vi "FTW-JSON-RegexHeader.vi"(1 "Regular Expression Body":string) -> (0 "Regular Expression with Header":string)   [LabVIEW 2014]
panel:
  # "Inputs"
  # "Outputs"
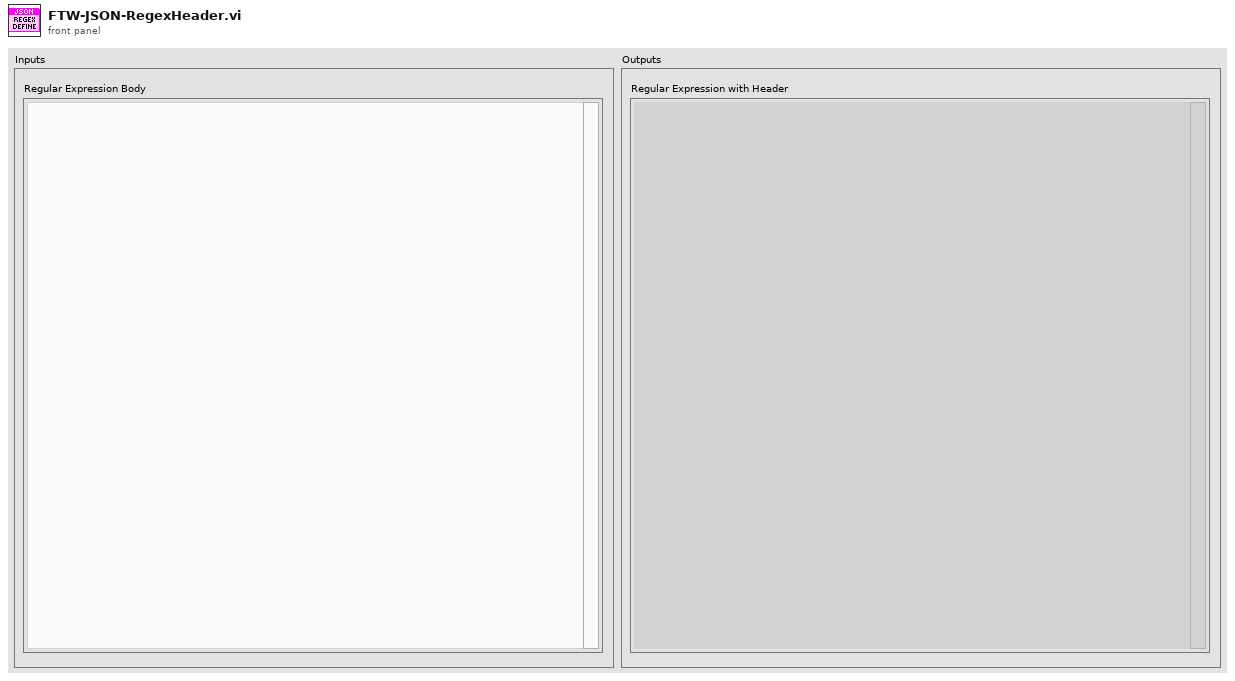
[diagram p1: front panel]
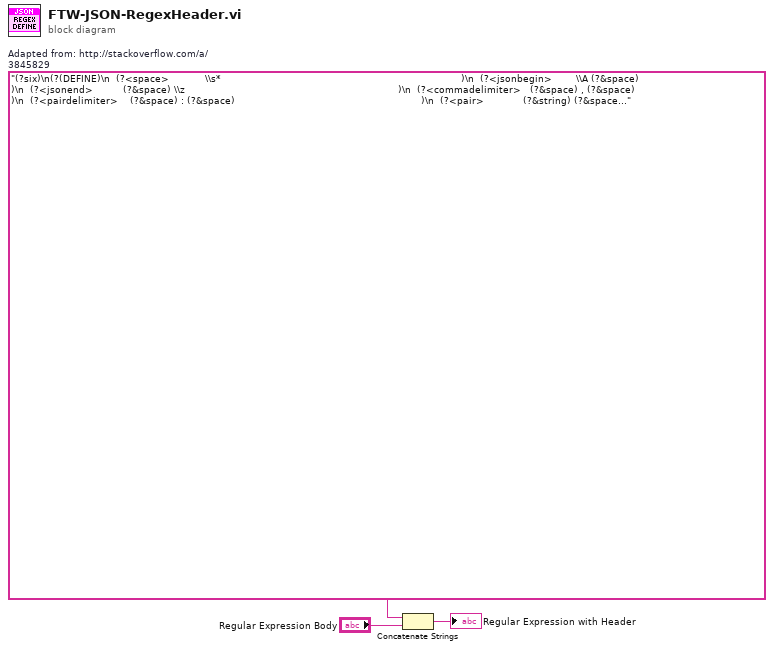
[diagram p0: block diagram]
diagram:
  w3 = "(?six)\n(?(DEFINE)\n  (?<space>            \\s*                                                                                )\n  (?<jsonbegin>        \\A (?&space)                                                                       )\n  (?<jsonend>          (?&space) \\z                                                                       )\n  (?<commadelimiter>   (?&space) , (?&space)                                                              )\n  (?<pairdelimiter>    (?&space) : (?&space)                                                              )\n  (?<pair>             (?&string) (?&space) : (?&space) (?&element)                                       )\n  (?<ftwpair>          (?&string) (?&space) : (?&space) (?&ftwelement)                                    )\n  (?<arrayelement>     (?&space) (?&element) (?&space)                                                    )\n  (?<number>           -? (?=[1-9]|0(?!\\d)) \\d+ (?:\\.\\d+)? (?:[eE][+-]?\\d+)?                              )\n  (?<ftwhexnum>        0x[0-9A-F]{2,16}                                                                   )\n  (?<boolean>          true | false                                                                       )\n  (?<null>             null                                                                               )\n  (?<stringinner>      (?:[^\"\\\\\\b\\f\\n\\r\\t] | \\\\[\"\\\\bfnrt\\/] | \\\\u[0-9a-f]{4})*                            )\n  (?<string>           \\\" (?&stringinner) \\\"                                                              )\n  (?<objectopen>       \\{ (?&space)                                                                       )\n  (?<arrayopen>        \\[ (?&space)                                                                       )\n  (?<objectclose>      (?&space) \\}                                                                       )\n  (?<arrayclose>       (?&space) \\]                                                                       )\n  (?<objectbegin>      (?&jsonbegin) (?&objectopen)                                                       )\n  (?<arraybegin>       (?&jsonbegin) (?&arrayopen)                                                        )\n  (?<objectend>        (?&objectclose) (?&jsonend)                                                        )\n  (?<arrayend>         (?&arrayclose)  (?&jsonend)                                                        )\n  (?<objectinner>      (?:(?&pair)    (?:(?&commadelimiter) (?&pair))*)?                                  )\n  (?<ftwobjectinner>   (?:(?&ftwpair) (?:(?&commadelimiter) (?&ftwpair))*)?                               )\n  (?<arrayinner>       (?:(?&arrayelement)(?:,(?&arrayelement))*)?                                        )\n  (?<array>            (?&arrayopen)  (?&arrayinner)  (?&arrayclose)                                      )\n  (?<object>           (?&objectopen) (?&objectinner) (?&objectclose)                                     )\n  (?<ftwobject>        (?&objectopen) (?&ftwobjectinner) (?&objectclose)                                  )\n  (?<element>          (?&number)|(?&boolean)|(?&string)|(?&array)|(?&object)|(?&null)                    )\n  (?<ftwelement>       (?&ftwhexnum)|(?&element)                                                          )\n  (?<validjson>        (?&jsonbegin) (?:(?&array)|(?&object)) (?&jsonend)                                 )\n)\n"  # Adapted from: http://stackoverflow.com/a/3845829
  n1 = Concatenate Strings(w3, "Regular Expression Body") -> (→"Regular Expression with Header":string)
